vi "split screen.vi"   [LabVIEW 2019, in "Tools.lvlib"]
uses:
  Tools.lvlib
  user32.dll
  LVWUtil32.dll
types:
  T1 = typedef "LVRectTypeDef.ctl" = cluster{"Left":i16, "Top":i16, "Right":i16, "Bottom":i16}
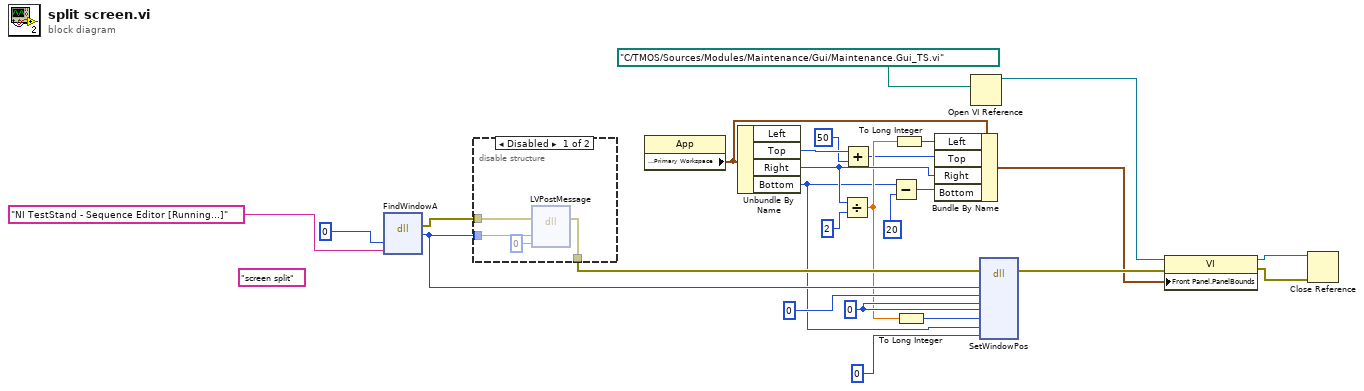
[diagram p0: block diagram]
diagram:
  (unwired) "screen split" ("arg2")
  w22 = 0 ("arg2")
  n1 = dll-call lib="user32.dll" fn="FindWindowA"("arg1"=0, "arg2"="NI TestStand - Sequence Editor [Running...]") -> (error out=w25:errorcluster, "return type"=w24:u32)  [unwired: 4 in, 2 out]
  n2 = disable-structure shown="Disabled" {
    disable-tunnel: w25 -> [w30 w31]
    disable-tunnel: w24 -> [w29 _]
    disable-tunnel: [w27 w31] -> w18
    frame Disabled {
      n3 = dll-call lib="C:/Projects/_Prywatne/MyCIT/Framework/Tools/screen split/LVWUtil32.DLL" fn="LVPostMessage"(error in=w30, "hWnd"=w29, "function"=u8 0) -> (error out=w27:errorcluster)  [unwired: 5 in, 1 out]
    }
    frame Enabled {
    }
  }
  n4 = property class="App"() -> ("Display:Primary Workspace"=w14:T1)  [unwired: 2 in, 2 out]
  n5 = Unbundle By Name(w14) -> ("Top"=w8:i16, "Right"=w13:i16, "Bottom"=w10:i16)  [unwired: 1 out]
  n6 = Divide(x=w13, y=i16 2) -> (x/y=w11:dbl)
  n7 = Add(x=w8, y=i16 50) -> (x+y=w6:i16)
  n8 = Subtract(x=w10, y=i16 20) -> (x-y=w5:i16)
  n9 = To Long Integer(number=w11) -> (32bit integer=w12:i32)
  n10 = To Long Integer(number=w11) -> (32bit integer=w19:i32)
  n11 = Bundle By Name(cluster=w14, "Left"=w12, "Top"=w6, "Right"=w13, "Bottom"=w5) -> (w9:T1)
  n12 = Open VI Reference(vi path=path "C:/TMOS/Sources/Modules/Maintenance/Gui/Maintenance.Gui_TS.vi") -> (vi reference=w15:refnum<vi>)  [unwired: 5 in, 1 out]
  n13 = dll-call lib="user32.dll" fn="SetWindowPos"(error in=w18, "arg1"=w24, "arg2"=0, "arg3"=w22, "arg4"=w22, "arg5"=w19, "arg7"=w10, "arg6"=u32 0) -> (error out=w16:errorcluster)  [unwired: 9 in, 2 out]
  n14 = property class="VI"(reference=w15, error in=w16, "Front Panel.PanelBounds"=w9) -> (reference out=w3:refnum<vi>, error out=w2:errorcluster)
  n15 = Close Reference(reference=w3, error in (no error)=w2) -> ()  [unwired: 1 out]
